vi "Use_AppBuilder_Cache.vi"(8 "error in (no error)":errorcluster, 11 "Build in":refnum<class "AB_PackedLibrary.lvclass">) -> (0 "error out":errorcluster, 2 "use cache":bool, 3 "Build out":refnum<class "AB_PackedLibrary.lvclass">)   [LabVIEW 2020, in "AB_PackedLibrary.lvclass"]
uses:
  <vilib>/AppBuilder/AB_Classes/PackedLib/AB_PackedLibrary.lvclass
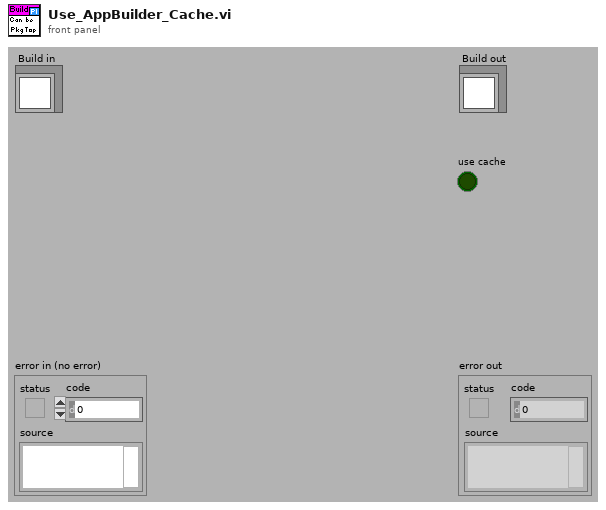
[diagram p1: front panel]
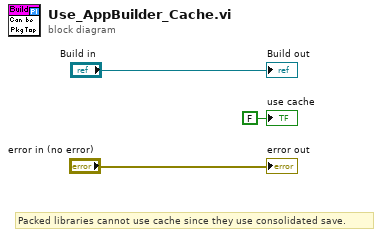
[diagram p0: block diagram]
diagram:
  # "Packed libraries cannot use cache since they use consolidated save."
  "error out" <- "error in (no error)"
  "Build out" <- "Build in"
  "use cache" <- FALSE ("use cache")
